vi "列表消息json处理.vi"(6 "error in (no error)":errorcluster caption="错误输入（无错误）", 7 "json input":string) -> (0 "error out":errorcluster caption="错误输出", 1 "top_stories":T1(array[cluster]), 2 "stories":T1(array[cluster]), 3 "date":string)   [LabVIEW 2012]
uses:
  <vilib>/addons/JSON API/JSON Value/JSON Value.lvclass
  <vilib>/addons/JSON API/JSON Value/Set from JSON string.vi
  <vilib>/addons/JSON API/Get Polymorphic/JSON GetSet.lvlib
  <vilib>/addons/JSON API/JSON Scalar/JSON Scalar.lvclass
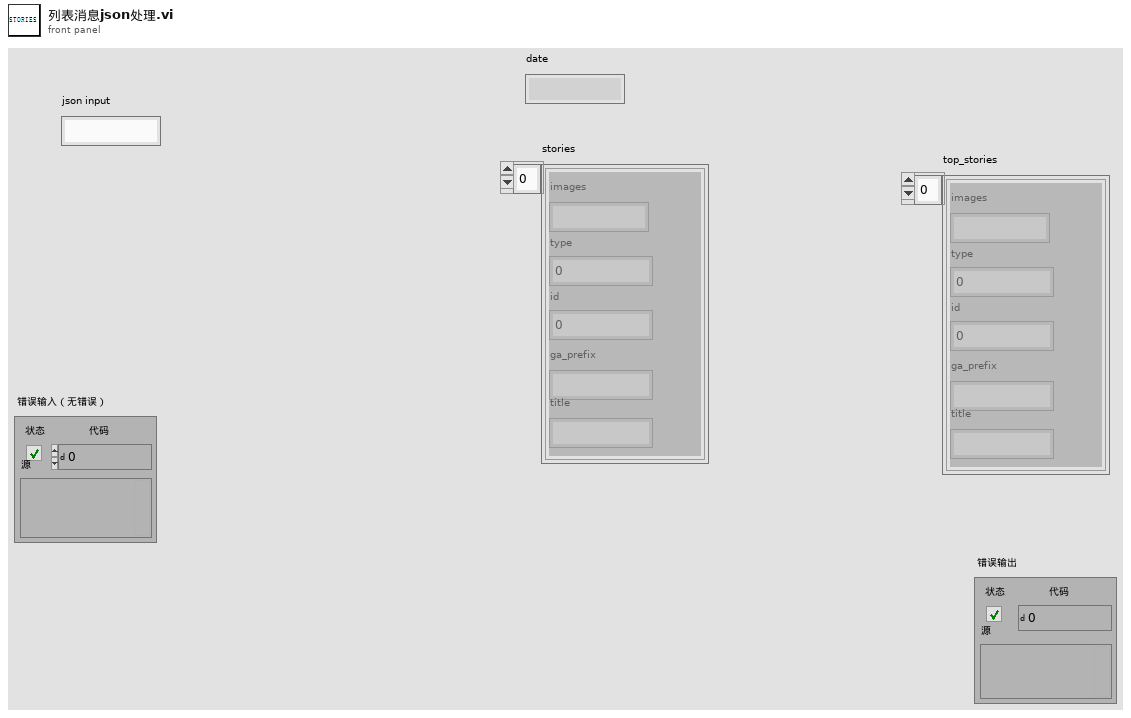
[diagram p1: front panel]
types:
  T1 = cluster{"images":string, "type":i32, "id":i64, "ga_prefix":string, "title":string}[]
  T2 = cluster{"LabVIEW Text":string, "Number":i32, "Number":i32, "LabVIEW Text":string, "LabVIEW Text":string}
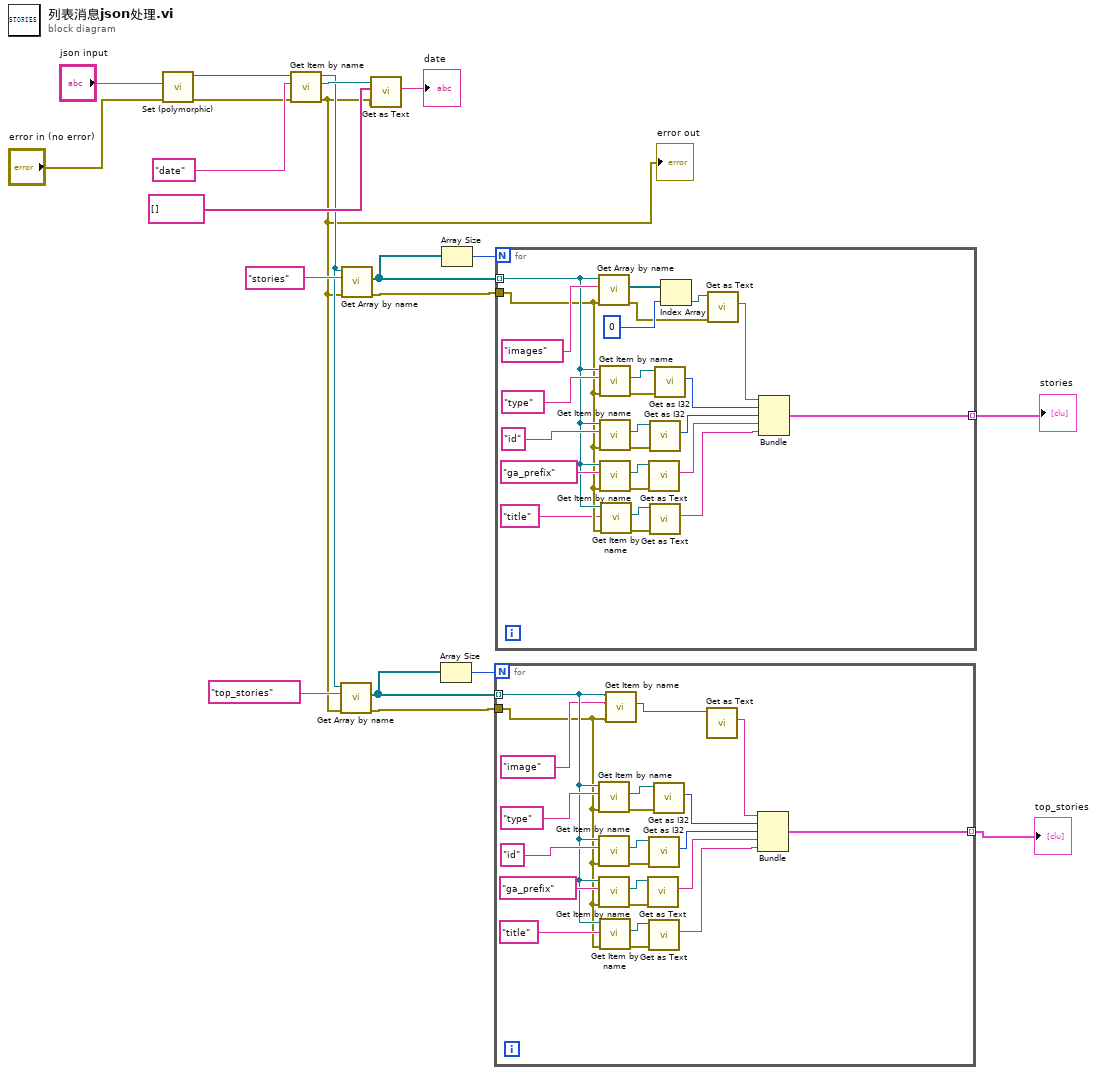
[diagram p0: block diagram]
diagram:
  n1 = call-poly <vilib>:"Set (polymorphic).vi"("error in (no error)"="error in (no error)", "JSON stream"="json input") -> ("error out"=w18:errorcluster, "JSON Value out"=w20:refnum<class "JSON Value.lvclass">)  [unwired: 7 in, 1 out]
  n2 = call-dynamic "Get Item by name.vi"("error in (no error)"=w18, "name"="date", "JSON Value In"=w20) -> ("error out"=w1:errorcluster, "Value"=w17:refnum<class "JSON Value.lvclass">, "JSON Value Out"=w4:refnum<class "JSON Value.lvclass">)  [unwired: 5 in, 1 out]
  "error out" <- w1
  n3 = call <vilib>:"Get Array by name.vi"("error in (no error)"=w1, "name"="top_stories", "JSON Value In"=w4) -> ("error out"=w5:errorcluster, "Array"=w6:refnum<class "JSON Value.lvclass">[])  [unwired: 5 in, 2 out]
  n4 = call <vilib>:"Get Array by name.vi"("error in (no error)"=w1, "name"="stories", "JSON Value In"=w4) -> ("error out"=w10:errorcluster, "Array"=w11:refnum<class "JSON Value.lvclass">[])  [unwired: 5 in, 2 out]
  n5 = call <vilib>:"Get as Text.vi"("error in (no error)"=w1, "Name Array"=string[] [], "JSON Scalar in"=w17) -> ("LabVIEW Text"=→"date":string)  [unwired: 6 in, 2 out]
  n6 = Array Size(array=w6) -> (size(s)=w7:i32)
  n7 = Array Size(array=w11) -> (size(s)=w12:i32)
  n8 = for {
    N: w7 -> [_]
    tunnel: w6 -> [w24] mode=indexing
    tunnel: w5 -> [w22]
    tunnel: [w25] -> w3 mode=indexing
    n9 = call-dynamic "Get Item by name.vi"("error in (no error)"=w22, "name"="type", "JSON Value In"=w24) -> ("error out"=w37:errorcluster, "Value"=w41:refnum<class "JSON Value.lvclass">)  [unwired: 5 in, 2 out]
    n10 = call-dynamic "Get Item by name.vi"("error in (no error)"=w22, "name"="id", "JSON Value In"=w24) -> ("error out"=w38:errorcluster, "Value"=w39:refnum<class "JSON Value.lvclass">)  [unwired: 5 in, 2 out]
    n11 = call-dynamic "Get Item by name.vi"("error in (no error)"=w22, "name"="ga_prefix", "JSON Value In"=w24) -> ("error out"=w34:errorcluster, "Value"=w35:refnum<class "JSON Value.lvclass">)  [unwired: 5 in, 2 out]
    n12 = call-dynamic "Get Item by name.vi"("error in (no error)"=w22, "name"="title", "JSON Value In"=w24) -> ("error out"=w31:errorcluster, "Value"=w32:refnum<class "JSON Value.lvclass">)  [unwired: 5 in, 2 out]
    n13 = call-dynamic "Get Item by name.vi"("error in (no error)"=w22, "name"="image", "JSON Value In"=w24) -> ("Value"=w21:refnum<class "JSON Value.lvclass">)  [unwired: 5 in, 3 out]
    n14 = call <vilib>:"Get as Text.vi"("error in (no error)"=w34, "JSON Scalar in"=w35) -> ("LabVIEW Text"=w27:string)  [unwired: 7 in, 2 out]
    n15 = call <vilib>:"Get as I32.vi"("error in (no error)"=w38, "JSON Scalar in"=w39) -> ("Number"=w28:i32)  [unwired: 7 in, 2 out]
    n16 = call <vilib>:"Get as Text.vi"("error in (no error)"=w31, "JSON Scalar in"=w32) -> ("LabVIEW Text"=w26:string)  [unwired: 7 in, 2 out]
    n17 = call <vilib>:"Get as I32.vi"("error in (no error)"=w37, "JSON Scalar in"=w41) -> ("Number"=w29:i32)  [unwired: 7 in, 2 out]
    n18 = call <vilib>:"Get as Text.vi"("JSON Scalar in"=w21) -> ("LabVIEW Text"=w30:string)  [unwired: 8 in, 2 out]
    n19 = Bundle("LabVIEW Text"=w30, "Number"=w29, "Number"=w28, "LabVIEW Text"=w27, "LabVIEW Text"=w26) -> (w25:T2)  [unwired: 1 in]
  }
  "top_stories" <- w3
  n20 = for {
    N: w12 -> [_]
    tunnel: w11 -> [w53] mode=indexing
    tunnel: w10 -> [w52]
    tunnel: [w43] -> w9 mode=indexing
    n21 = call <vilib>:"Get Array by name.vi"("error in (no error)"=w52, "name"="images", "JSON Value In"=w53) -> ("error out"=w57:errorcluster, "Array"=w66:refnum<class "JSON Value.lvclass">[])  [unwired: 5 in, 2 out]
    n22 = call-dynamic "Get Item by name.vi"("error in (no error)"=w52, "name"="type", "JSON Value In"=w53) -> ("error out"=w58:errorcluster, "Value"=w62:refnum<class "JSON Value.lvclass">)  [unwired: 5 in, 2 out]
    n23 = call-dynamic "Get Item by name.vi"("error in (no error)"=w52, "name"="id", "JSON Value In"=w53) -> ("error out"=w59:errorcluster, "Value"=w60:refnum<class "JSON Value.lvclass">)  [unwired: 5 in, 2 out]
    n24 = call-dynamic "Get Item by name.vi"("error in (no error)"=w52, "name"="ga_prefix", "JSON Value In"=w53) -> ("error out"=w54:errorcluster, "Value"=w55:refnum<class "JSON Value.lvclass">)  [unwired: 5 in, 2 out]
    n25 = call-dynamic "Get Item by name.vi"("error in (no error)"=w52, "name"="title", "JSON Value In"=w53) -> ("error out"=w49:errorcluster, "Value"=w50:refnum<class "JSON Value.lvclass">)  [unwired: 5 in, 2 out]
    n26 = call <vilib>:"Get as Text.vi"("error in (no error)"=w54, "JSON Scalar in"=w55) -> ("LabVIEW Text"=w45:string)  [unwired: 7 in, 2 out]
    n27 = call <vilib>:"Get as I32.vi"("error in (no error)"=w59, "JSON Scalar in"=w60) -> ("Number"=w46:i32)  [unwired: 7 in, 2 out]
    n28 = call <vilib>:"Get as Text.vi"("error in (no error)"=w49, "JSON Scalar in"=w50) -> ("LabVIEW Text"=w44:string)  [unwired: 7 in, 2 out]
    n29 = call <vilib>:"Get as I32.vi"("error in (no error)"=w58, "JSON Scalar in"=w62) -> ("Number"=w47:i32)  [unwired: 7 in, 2 out]
    n30 = Index Array(array=w66, index=0) -> (element=w64:refnum<class "JSON Value.lvclass">)
    n31 = call <vilib>:"Get as Text.vi"("error in (no error)"=w57, "JSON Scalar in"=w64) -> ("LabVIEW Text"=w48:string)  [unwired: 7 in, 2 out]
    n32 = Bundle("LabVIEW Text"=w48, "Number"=w47, "Number"=w46, "LabVIEW Text"=w45, "LabVIEW Text"=w44) -> (w43:T2)  [unwired: 1 in]
  }
  "stories" <- w9
